vi "Write Receive Only.vi"(8 "error in (no error)":errorcluster, 10 "Receive Only":bool, 11 "View Actor in":refnum<class "View Actor.lvclass">) -> (0 "error out":errorcluster, 3 "View Actor out":refnum<class "View Actor.lvclass">)   [LabVIEW 2016, in "Event Actors.lvlib" / "View Actor.lvclass"]
uses:
  View Actor.lvclass
  View Actor.lvclass/View Actor.ctl
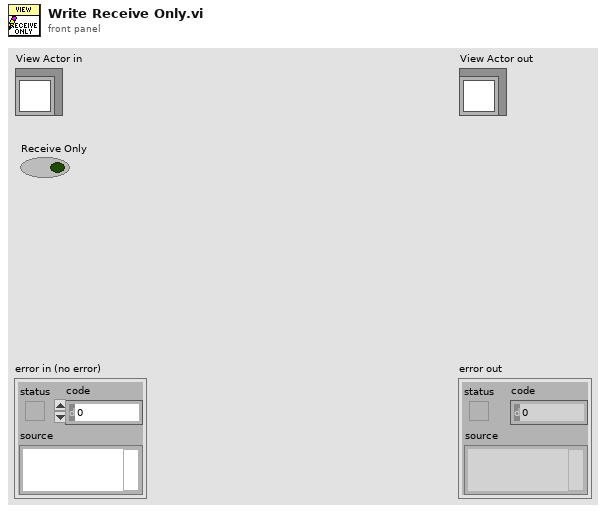
[diagram p1: front panel]
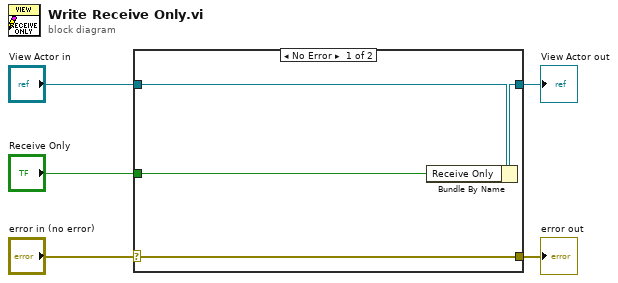
[diagram p0: block diagram]
diagram:
  n1 = case shown="No Error" "error in (no error)" {
    selector: "error in (no error)" -> [w9 w10]
    tunnel: [w9 w10] -> w4
    tunnel: [w7 w11] -> w2
    tunnel: "View Actor in" -> [w8 w11]
    tunnel: "Receive Only" -> [w6 _]
    frame No Error {
      n2 = Bundle By Name(cluster=w8, "Receive Only"=w6) -> (w7:refnum<class "View Actor.lvclass">)
    }
    frame Error {
    }
  }
  "error out" <- w4
  "View Actor out" <- w2
